vi "Aquisicao.vi"() -> ()   [LabVIEW 2020]
uses:
  <vilib>/Analysis/baseanly.llb/Mean (DBL).vi
  <vilib>/Analysis/NI_AALBase.lvlib
panel:
  in  "stop":bool
  in  "rate":dbl=100.0
  out "mean":dbl=2.8624583478545538 format="%0.4f"
  in  "Write File?":bool=TRUE
  in  "Filename":string="exp1.txt"
  out "Waveform Graph":dbl[](graph)=[2.9147608995839254, 2.919454134157277, 2.9244012330140685, 2.9285314096254296, 2.93140853817109, 2.931206748612458, 2.9272881255706307, 2.918594901197939, 2.904974105990259, 2.8860644715442323, 2.8624583478545538]
  in  "stop (F)":bool
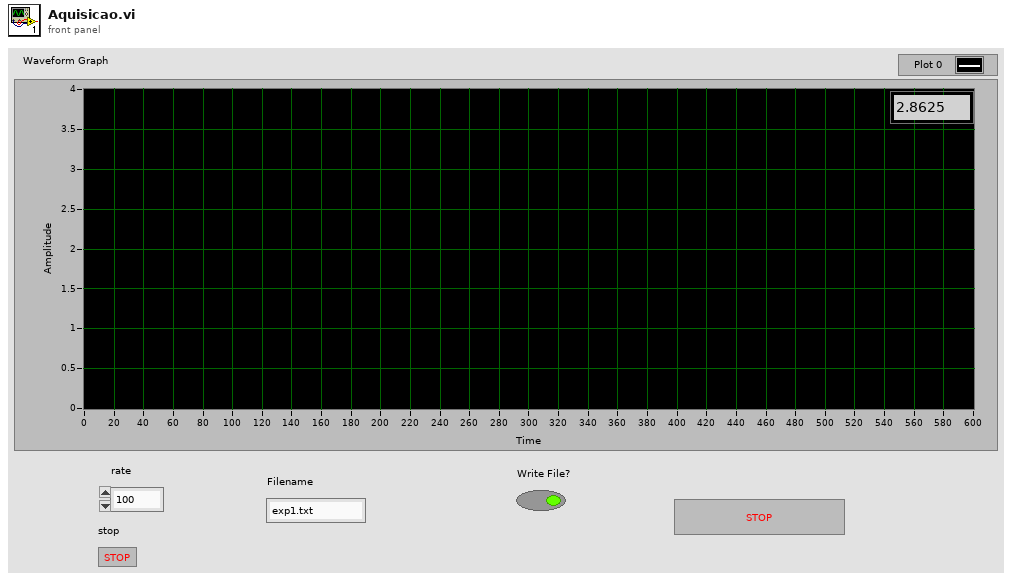
[diagram p1: front panel]
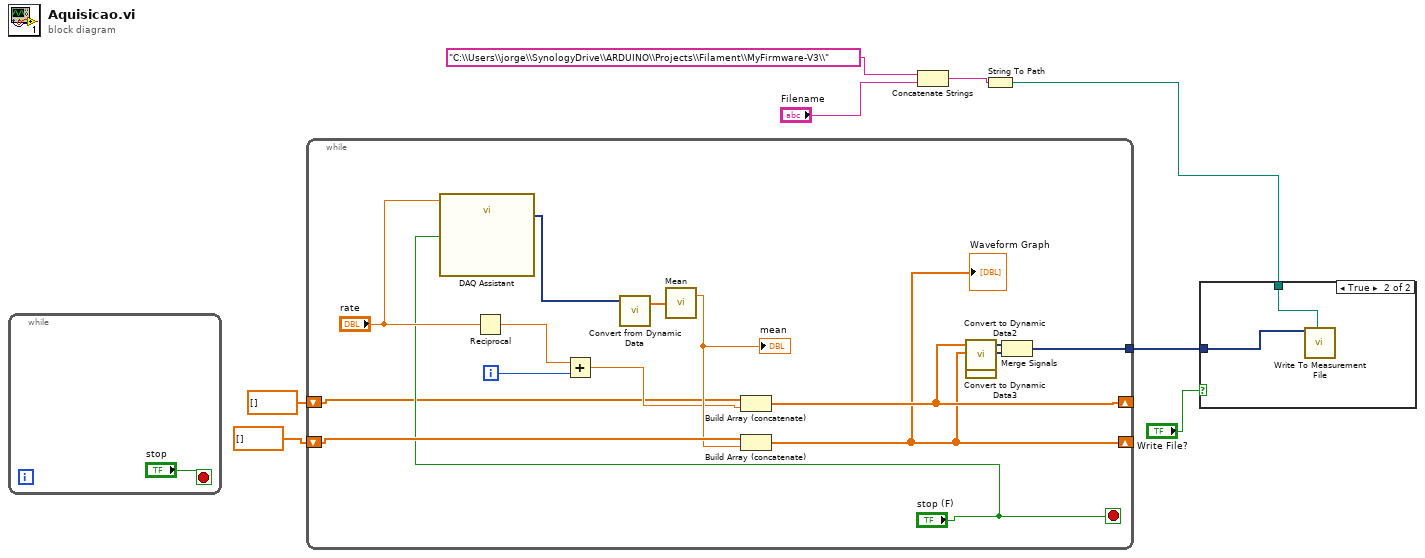
[diagram p0: block diagram]
diagram:
  n1 = while {
    stop <- "stop" stop-if-true
  }
  n2 = while {
    shift-right: [w12] -> _
    shift-left: dbl[] [] -> [w23]
    shift-right: [w14] -> _
    shift-left: dbl[] [] -> [w15]
    tunnel: [w10] -> w1
    i -> [w17]
    stop <- "stop (F)" stop-if-true
    n3 = call "DAQ Assistant"("rate"="rate", "stop (F)"="stop (F)") -> ("data"=w22:dynamicdata)  [unwired: 14 in, 3 out]
    n4 = Reciprocal(x="rate") -> (1/x=w18:dbl)
    n5 = Add(x=w18, y=w17) -> (x+y=w16:dbl)
    n6 = call "Convert from Dynamic Data"("Dynamic Data Type"=w22) -> ("Array"=w24:dbl[])  [unwired: 3 in]
    n7 = call-poly <vilib>:"Mean.vi"("X"=w24) -> ("mean"=w20:dbl)  [unwired: 1 out]
    "mean" <- w20
    n8 = Build Array (concatenate)(w15, w16) -> (w14:dbl[])
    n9 = Build Array (concatenate)(w23, w20) -> (w12:dbl[])
    "Waveform Graph" <- w12
    n10 = call "Convert to Dynamic Data2"("Array"=w14) -> ("Dynamic Data Type"=w13:dynamicdata)  [unwired: 3 in]
    n11 = call "Convert to Dynamic Data3"("Array"=w12) -> ("Dynamic Data Type"=w11:dynamicdata)  [unwired: 3 in]
    n12 = Merge Signals(w13, w11) -> (w10:dynamicdata)
  }
  n13 = Concatenate Strings("C:\\Users\\jorge\\SynologyDrive\\ARDUINO\\Projects\\Filament\\MyFirmware-V3\\", "Filename") -> (w5:string)
  n14 = String To Path(string=w5) -> (path=w4:path)
  n15 = case shown="True" "Write File?" {
    tunnel: w4 -> [_ w26]
    tunnel: w1 -> [_ w25]
    frame False {
    }
    frame True {
      n16 = call "Write To Measurement File"("Signals"=w25, "Filename"=w26) -> ()  [unwired: 15 in, 3 out]
    }
  }
